vi "Get Object to File (Sequential).vi"(4 "Region":T1, 6 "Version ID":string, 7 "Chunk size (kB)":i32=1024 min=1024, 8 "error in (no error)":errorcluster, 9 "Bucket":string, 10 "Object Path":string, 11 "File path":path) -> (0 "error out":errorcluster)   [LabVIEW 2015, in "LV Interface for Amazon S3.lvlib"]
doc: "This operation <B>retrieves an object</B> from Amazon S3 <B>to a file</B>. The operation <B>retrieves object data in chunks</B>. You <B>must have READ access</B> to the object. If you grant READ access to the anonymous user, you can return the object without using an authorization header. To distribute large files to many people, you can <B>save bandwidth costs using BitTorrent</B>."
uses:
  LV Interface for Amazon S3.lvlib
  Typedefs/AMZ_S3_LocationConstraint.ctl
  Typedefs/AMZ_S3_API_GET Object Request Parameters.ctl
  Typedefs/AMZ_S3_API_GET Request Range.ctl
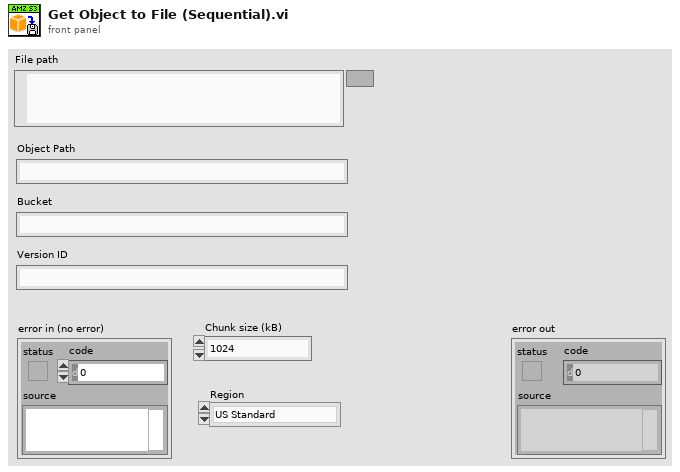
[diagram p1: front panel]
types:
  T1 = typedef "LV Interface for Amazon S3.lvlib/AMZ_S3_LocationConstraint.ctl" = enum16{"US Standard", "us-east-2", "us-west-1", "us-west-2", "ap-northeast-1", "ap-northeast-2", "ap-southeast-1", "ap-southeast-2", "ca-central-1", "eu-central-1", "eu-west-1", "eu-west-2", "sa-east-1"}
  T2 = enum16{"open", "replace", "create", "open or create", "replace or create", "replace or create with confirmation"}
  T3 = typedef "LV Interface for Amazon S3.lvlib/AMZ_S3_API_GET Object Request Parameters.ctl" = cluster{"Range":T4, "If Modified Since":timestamp, "If Unmodified Since":timestamp, "Matching ETag":string, "Nonmatching ETag":string}
  T4 = typedef "LV Interface for Amazon S3.lvlib/AMZ_S3_API_GET Request Range.ctl" = cluster{"Start":i64, "Length":i64}
  T5 = typedef "LV Interface for Amazon S3.lvlib/AMZ_S3_API_GETObjectResult.ctl" = cluster{"Content Length (bytes)":u64, "Content Type":string, "ETag":string, "Delete marker":bool, "Version ID":string, "Object Size (bytes)":u64}
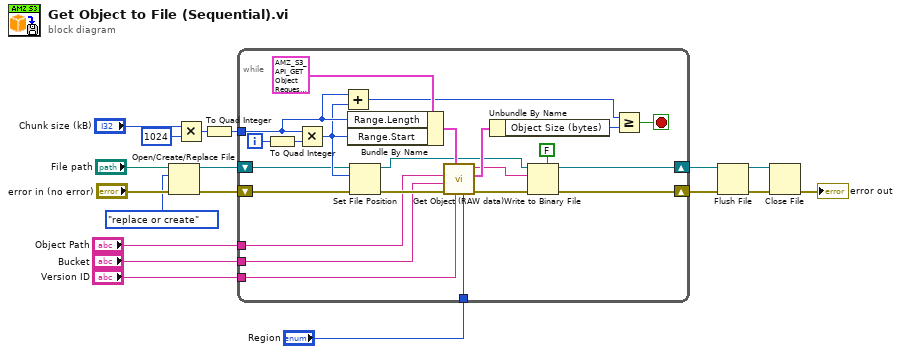
[diagram p0: block diagram]
diagram:
  n1 = Open/Create/Replace File(file path (use dialog)="File path", error in="error in (no error)", operation (0:open)=T2."replace or create") -> (refnum out=w15:refnum<file>, error out=w14:errorcluster)  [unwired: 3 in, 1 out]
  n2 = Multiply(x="Chunk size (kB)", y=1024) -> (x*y=w3:i32)
  n3 = To Quad Integer(1:w3) -> (0:w2:i64)
  n4 = while {
    tunnel: w2 -> [w22]
    tunnel: "Object Path" -> [w33]
    tunnel: "Bucket" -> [w32]
    shift-right: [w27] -> w10
    shift-left: w15 -> [w20]
    shift-right: [w28] -> w11
    shift-left: w14 -> [w35]
    tunnel: "Version ID" -> [w26]
    tunnel: "Region" -> [w19]
    i -> [w24]
    stop <- w36 stop-if-true
    n5 = To Quad Integer(1:w24) -> (0:w23:i64)
    n6 = Multiply(x=w22, y=w23) -> (x*y=w21:i64)
    n7 = Add(x=w22, y=w21) -> (x+y=w37:i64)
    n8 = Bundle By Name(cluster=T3 {"Range"={"Start"=0, "Length"=0}, "If Modified Since"=timestamp(0 s since 1904-01-01), "If Unmodified Since"=timestamp(0 s since 1904-01-01), "Matching ETag"="", "Nonmatching ETag"=""} ("Request Parameters"), "Range.Length"=w22, "Range.Start"=w21) -> (w40:T3)
    n9 = Set File Position(offset (in bytes) (0)=w21, refnum=w20, error in=w35) -> (refnum out=w29:refnum<file>, error out=w34:errorcluster)  [unwired: 1 in]
    n10 = call "Get Object (RAW data).vi"("Region"=w19, "Version ID"=w26, "Request Parameters"=w40, "error in (no error)"=w34, "Bucket"=w32, "Object Path"=w33) -> ("error out"=w31:errorcluster, "GetObjectResult"=w39:T5, "Data"=w30:string)  [unwired: 3 in]
    n11 = Unbundle By Name(w39) -> ("Object Size (bytes)"=w38:u64)
    n12 = Write to Binary File(file (use dialog)=w29, data=w30, error in=w31, 5:FALSE ("prepend array or string size? (T)")) -> (refnum out=w27:refnum<file>, error out=w28:errorcluster)  [unwired: 2 in, 1 out]
    n13 = Greater Or Equal?(x=w37, y=w38) -> (x >= y?=w36:bool)
  }
  n14 = Flush File(refnum=w10, error in=w11) -> (refnum out=w8:refnum<file>, error out=w9:errorcluster)
  n15 = Close File(refnum=w8, error in=w9) -> (error out=→"error out":errorcluster)  [unwired: 1 out]
